vi "Hide Charm.vi"(8 "error in (no error)":errorcluster, 10 "Stop Charm? (T)":bool=TRUE, 11 "MainController in":refnum<class "MainController.lvclass">) -> (0 "error out":errorcluster, 3 "MainController out":refnum<class "MainController.lvclass">)   [LabVIEW 2012, in "Win8uiFramework.lvlib" / "MainController.lvclass"]
uses:
  MainController.lvclass
  MainController.lvclass/MainController.ctl
  Visibility Direction.ctl
  Visiblity States.ctl
  <vilib>/ActorFramework/Message Enqueuer/Message Enqueuer.lvclass/Message Enqueuer.ctl
  <vilib>/ActorFramework/Message Enqueuer/Message Enqueuer.lvclass
  Write Charm Enqueuer.vi
  Write Charm State.vi
  Read Charm Enqueuer.vi
  Read Charm State.vi
  <vilib>/ActorFramework/Message Enqueuer/Enqueue.vi
  <vilib>/ActorFramework/Message Priority Queue/Priority Enqueue.vi
  Remove From SubPanel Msg.lvclass
  <vilib>/ActorFramework/Stop Msg/Stop Msg.lvclass
  Win8uiFramework.lvlib
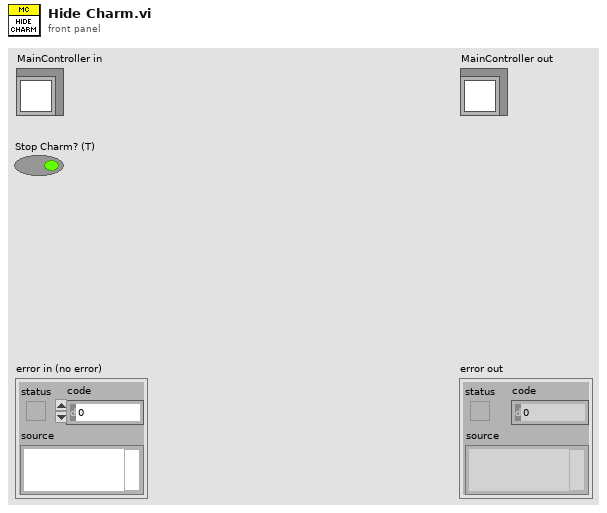
[diagram p1: front panel]
types:
  T1 = typedef "Win8uiFramework.lvlib/Visibility Direction.ctl" = enum16{"Show", "Hide"}
  T2 = typedef "Win8uiFramework.lvlib/MainController.lvclass/Visiblity States.ctl" = enum16{"Disabled", "Hidden - Unpopulated", "Hidden - Populated", "Visible"}
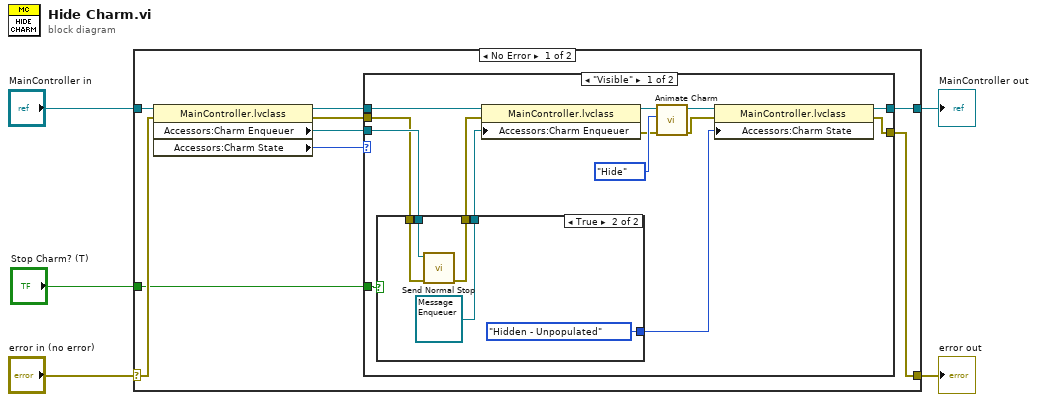
[diagram p0: block diagram]
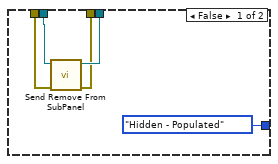
[diagram p2: hidden frame]
diagram:
  n1 = case shown="No Error" "error in (no error)" {
    selector: "error in (no error)" -> [w12 w42]
    tunnel: [w9 w42] -> w4
    tunnel: [w8 w41] -> w2
    tunnel: "MainController in" -> [w14 w41]
    tunnel: "Stop Charm? (T)" -> [w10 _]
    frame No Error {
      n2 = property class="MainController.lvclass"(reference=w14, error in=w12) -> (reference out=w13:refnum<class "MainController.lvclass">, error out=w11:errorcluster, "Accessors:Charm Enqueuer"=w7:refnum<class "Message Enqueuer.lvclass">, "Accessors:Charm State"=w6:T2)
      n3 = case shown="\"Visible\"" w6 {
        tunnel: w13 -> [w28 w40]
        tunnel: w7 -> [w27 _]
        tunnel: w11 -> [w26 w39]
        tunnel: w10 -> [w23 _]
        tunnel: [w16 w39] -> w9
        tunnel: [w18 w40] -> w8
        frame "Visible" {
          n4 = case shown="True" w23 {
            tunnel: w27 -> [w33 w38]
            tunnel: w26 -> [w32 w37]
            tunnel: [w30 w36] -> w25
            tunnel: [w31 refnum<class "Message Enqueuer.lvclass"> refnum ("AppBar Enqueuer")] -> w24
            tunnel: [Visiblity_States."Hidden - Populated" ("Charm State") Visiblity_States."Hidden - Unpopulated" ("Charm State")] -> w15
            frame False {
              n5 = call "Send Remove From SubPanel.vi"("error in (no error)"=w32, "Message Enqueuer"=w33) -> ("error out"=w30:errorcluster, "Message Enqueuer out"=w31:refnum<class "Message Enqueuer.lvclass">)  [unwired: 8 in]
            }
            frame True {
              n6 = call <vilib>:"Send Normal Stop.vi"("error in (no error)"=w37, "Message Enqueuer"=w38) -> ("error out"=w36:errorcluster)  [unwired: 9 in]
            }
          }
          n7 = property class="MainController.lvclass"(reference=w28, error in=w25, "Accessors:Charm Enqueuer"=w24) -> (reference out=w22:refnum<class "MainController.lvclass">, error out=w20:errorcluster)
          n8 = call-dynamic "Animate Charm.vi"("error in (no error)"=w20, "Direction"=Visibility_Direction."Hide", "MainController in"=w22) -> ("error out"=w17:errorcluster, "MainController out"=w19:refnum<class "MainController.lvclass">)  [unwired: 7 in]
          n9 = property class="MainController.lvclass"(reference=w19, error in=w17, "Accessors:Charm State"=w15) -> (reference out=w18:refnum<class "MainController.lvclass">, error out=w16:errorcluster)
        }
        frame "Disabled".."Hidden - Populated" {
          # "No charm visible, ignore hide request."
        }
      }
    }
    frame Error {
    }
  }
  "error out" <- w4
  "MainController out" <- w2
